vi "Rotation Control.vi"(11 "Color Sensor Input":string) -> (3 "Done":bool)   [LabVIEW 2019]
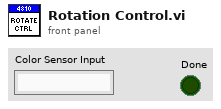
[diagram p1: front panel]
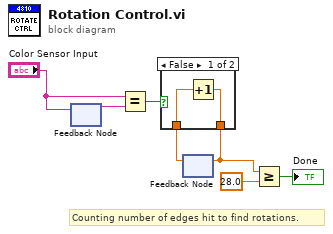
[diagram p0: block diagram]
diagram:
  # "Counting number of edges hit to find rotations."
  n1 = feedback-in #1("Color Sensor Input") -> ()
  n2 = feedback #1() -> (w7:string)  [unwired: 1 in]
  n3 = Equal?(x="Color Sensor Input", y=w7) -> (x = y?=w5:bool)
  n4 = feedback #2() -> (w4:dbl)  [unwired: 1 in]
  n5 = case shown="False" w5 {
    tunnel: [w9 w10] -> w3
    tunnel: w4 -> [w8 w10]
    frame False {
      n6 = Increment(x=w8) -> (x+1=w9:dbl)
    }
    frame True {
    }
  }
  n7 = feedback-in #2(w3) -> ()
  n8 = Greater Or Equal?(x=w3, y=28.0) -> (x >= y?=→"Done":bool)
